vi "UIRef.vi"(8 "error in":errorcluster, 11 "Systems in":refnum<class "Systems.lvclass">) -> (0 "error out":errorcluster, 2 "VI refnum":refnum<vi>, 3 "Systems out":refnum<class "Systems.lvclass">)   [LabVIEW 2013, in "PL Framework Configuration Tool.lvlib" / "Systems.lvclass"]
doc: "Stores the static reference to the UI of the node."
uses:
  Systems.lvclass
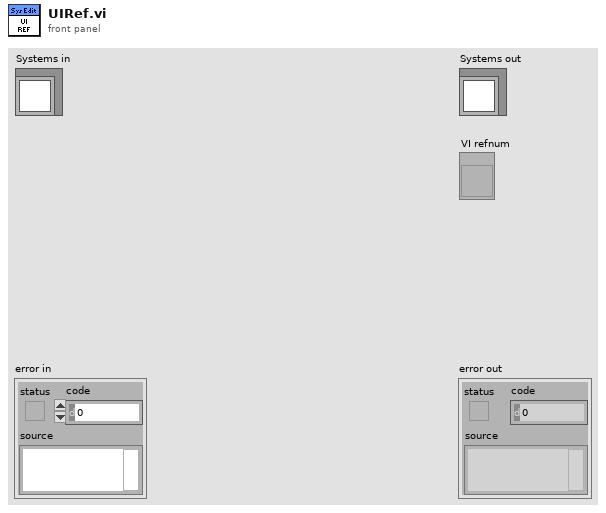
[diagram p1: front panel]
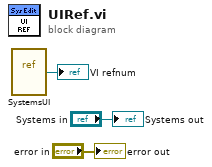
[diagram p0: block diagram]
diagram:
  n1 = vi-ref "SystemsUI.vi"() -> (→"VI refnum":refnum<vi>)
  "error out" <- "error in"
  "Systems out" <- "Systems in"
